vi "SetState.vi"(8 "Error In":errorcluster, 10 "State":bool, 11 "reference in":refnum<class "VdDigitalControl.lvclass">) -> (0 "Error Out":errorcluster, 3 "reference in":refnum<class "VdDigitalControl.lvclass">)   [LabVIEW 2020, in "VdDigitalControl.lvclass"]
uses:
  VdDigitalControl.lvclass
  VdDigitalControl.lvclass/VdDigitalControl.ctl
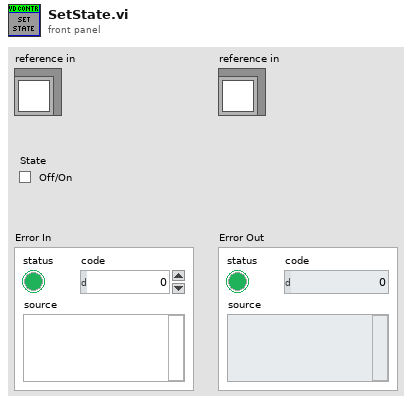
[diagram p1: front panel]
types:
  T1 = typedef "VdDigitalControl.lvclass/ObjectAttributes.ctl" = cluster{"CurrentState":bool}
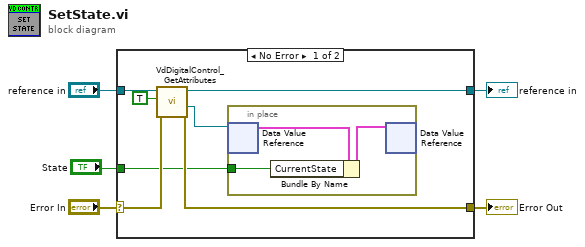
[diagram p0: block diagram]
diagram:
  n1 = case shown="No Error" "Error In" {
    selector: "Error In" -> [w12 w17]
    tunnel: [w11 w17] -> w4
    tunnel: [w9 w16] -> w2
    tunnel: "reference in" -> [w10 w16]
    tunnel: "State" -> [w7 _]
    frame No Error {
      n2 = call "VdDigitalControl_GetAttributes.vi"("error in"=w12, "OnlyGetDvrReference(False)"=TRUE, "reference in"=w10) -> ("error out"=w11:errorcluster, "DataRef"=w8:refnum<data-value>, "reference out"=w9:refnum<class "VdDigitalControl.lvclass">)  [unwired: 5 in, 1 out]
      n3 = in-place {
        in-place-border: w7 -> [w13]
        n4 = in-place-dvr #1(w8) -> (w15:T1)  [unwired: 1 out]
        n5 = Bundle By Name(cluster=w15, "CurrentState"=w13) -> (w14:T1)
        n6 = in-place-dvr #1(w14) -> ()  [unwired: 2 out]
      }
    }
    frame Error {
    }
  }
  "Error Out" <- w4
  "reference in" <- w2
